vi "fgv_950_parsing-arr.vi"(7 "cmd":T1, 11 "950 parsing arr":cluster{"950-arr 1":dbl[], "950-arr 2":dbl[]}) -> (3 "950 parsing arr 2":cluster{"950-arr 1":dbl[], "950-arr 2":dbl[]})   [LabVIEW 2019]
uses:
  _ctrl/rw.ctl
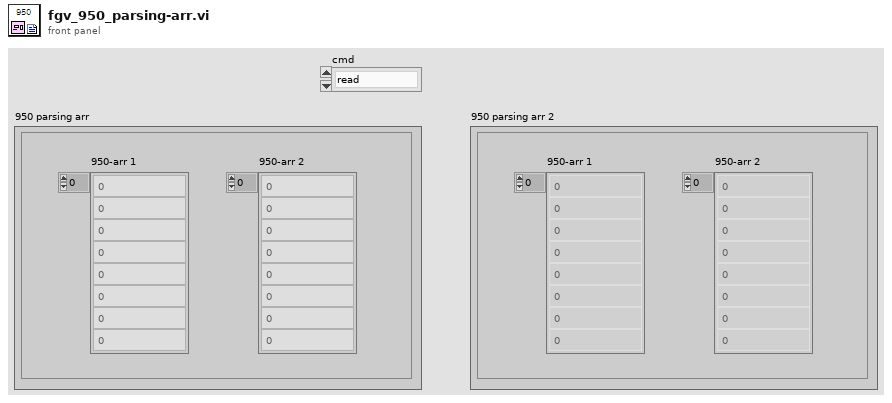
[diagram p1: front panel]
types:
  T1 = typedef "rw.ctl" = enum16{"read", "write"}
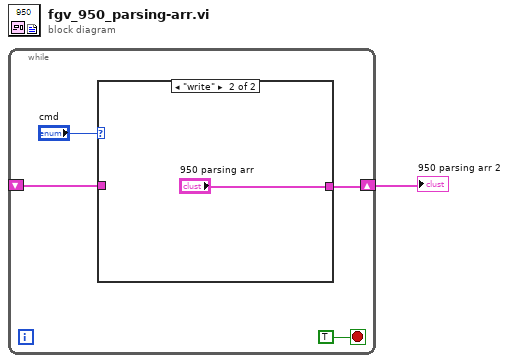
[diagram p0: block diagram]
diagram:
  n1 = while {
    shift-right: [w3] -> w1
    shift-left: _ -> [w2]
    stop <- TRUE stop-if-true
    n2 = case shown="\"write\"" "cmd" {
      tunnel: [w6 "950 parsing arr"] -> w3
      tunnel: w2 -> [w6 _]
      frame "read", Default {
      }
      frame "write" {
      }
    }
  }
  "950 parsing arr 2" <- w1
